vi "Initialize.vi"(5 "Config Path":path, 7 "VI Reference":refnum<vi>, 8 "error in (no error)":errorcluster, 11 "ControlValues in":refnum<class "ControlValues.lvclass">) -> (0 "error out":errorcluster, 3 "ControlValues out":refnum<class "ControlValues.lvclass">)   [LabVIEW 2016, in "ControlValues.lvclass"]
uses:
  ControlValues.lvclass
  ControlValues.lvclass/ControlValues.ctl
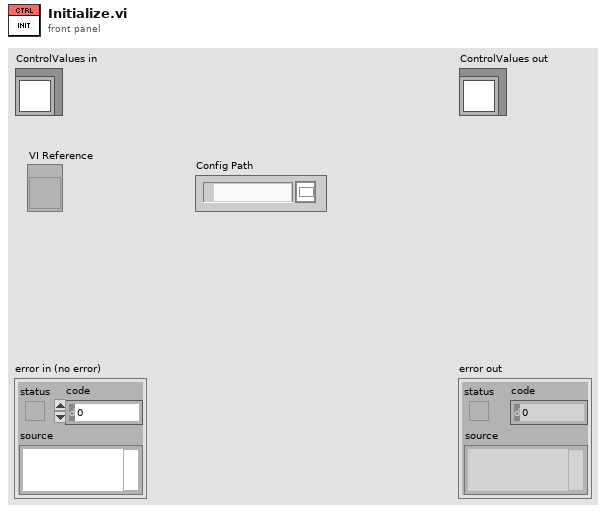
[diagram p1: front panel]
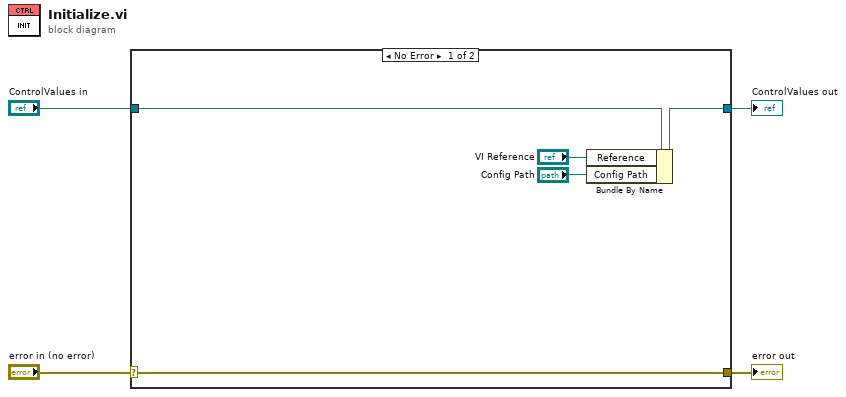
[diagram p0: block diagram]
diagram:
  n1 = case shown="No Error" "error in (no error)" {
    selector: "error in (no error)" -> [w9 w11]
    tunnel: [w9 w11] -> w3
    tunnel: [w7 w10] -> w1
    tunnel: "ControlValues in" -> [w8 w10]
    frame No Error {
      n2 = Bundle By Name(cluster=w8, "Reference"="VI Reference", "Config Path"="Config Path") -> (w7:refnum<class "ControlValues.lvclass">)
    }
    frame Error {
    }
  }
  "error out" <- w3
  "ControlValues out" <- w1
